vi "to_map.from_cluster_pairs.vi"(10 "properties (cluster pairs)":cluster{"name":string, "value":string}[](array[cluster])) -> (2 "properties (map)":map{string, string}(c390))   [LabVIEW 2020, in "nominal types.lvlib" / "properties.lvclass"]
uses:
  properties.lvclass
  properties.lvclass/properties.ctl
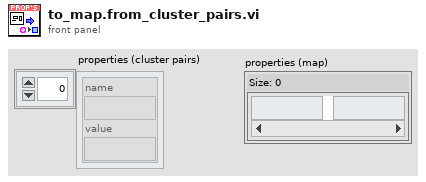
[diagram p1: front panel]
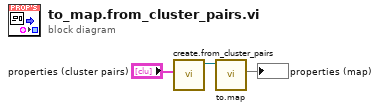
[diagram p0: block diagram]
diagram:
  n1 = call "create.from_cluster_pairs.vi"("properties"="properties (cluster pairs)") -> ("properties out"=w3:refnum<class "properties.lvclass">)  [unwired: 10 in]
  n2 = call "to.map.vi"("properties in"=w3) -> ("properties"=→"properties (map)":map{string, string})  [unwired: 8 in, 2 out]
